vi "Hardware Module.vi"(4 "Light intensity [%]":dbl(ramp), 5 "Mode":enum16{"Ohm", "DcV"}(ring), 6 "write buffer":string, 7 "State":T1(ring), 8 "error in (no error)":errorcluster, 9 "byte count":u32, 10 "baud rate (9600)":u32=9600, 11 "VISA resource name":refnum<visa-resource-name>) -> (0 "error out":errorcluster, 1 "return count":u32, 2 "read buffer":string, 3 "VISA resource name out":refnum<visa-resource-name>)   [LabVIEW 2019]
doc: "Funkcja służy do komunikacji za pomocą portu szeregowergo z multimetrem cyfrowym SANWA PC5000a. Komunikacja odbywa się poprzez bibliotekę NI-VISA z wykorzystaniem podstawowych funkcji portu szeregowego. Funkcja umożliwia emulację hardwaru wówczas jako nazwę urządzenia podać: VirtualDevice1\n\n- VISA resource name specifies the resource to be opened.\n- baud rate is the rate of transmission. The default is 9600. \n- write buffer contains the data to be written to the device. \n- return count contains the actual number of bytes written. \n- State defines the functionality of the function. It contains three values Configure Port, Write, Read and Close\n- Light intensity [%] is used during emulation.\n- error out contains error information. This output provides standard error out functionality.\n\nWięcej pomocy można znaleźć w pomocy funkcji:\nVISA Configure Serial Port VI \nVISA Write Function\nVISA Read Function"
uses:
  <vilib>/Instr/_visa.llb/VISA Configure Serial Port (Instr).vi
  <vilib>/ptbypt/NI_PtbyPt.lvlib
panel:
  # "Inputs"
  # "Outputs"
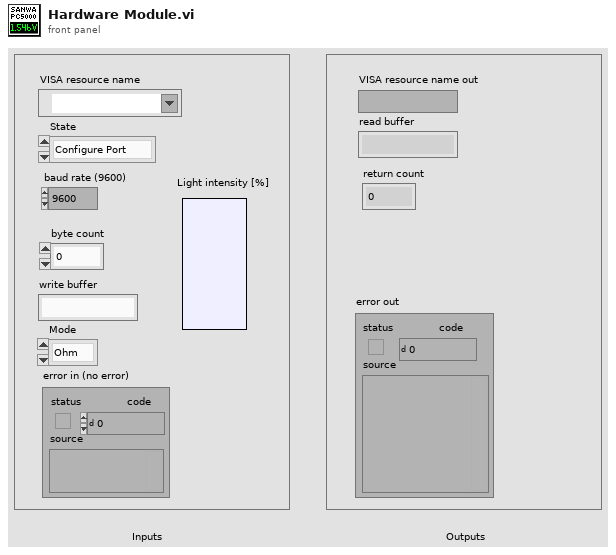
[diagram p1: front panel]
types:
  T1 = enum16{"Configure Port", "Write", "Read", "Close"}
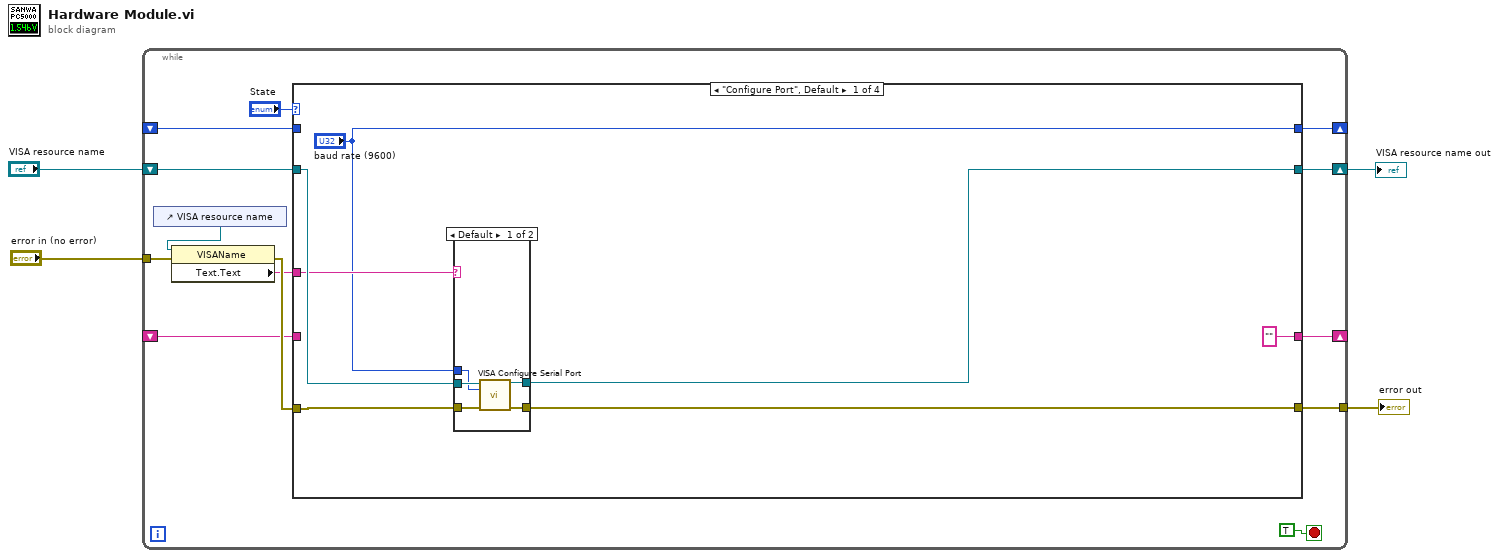
[diagram p0: block diagram]
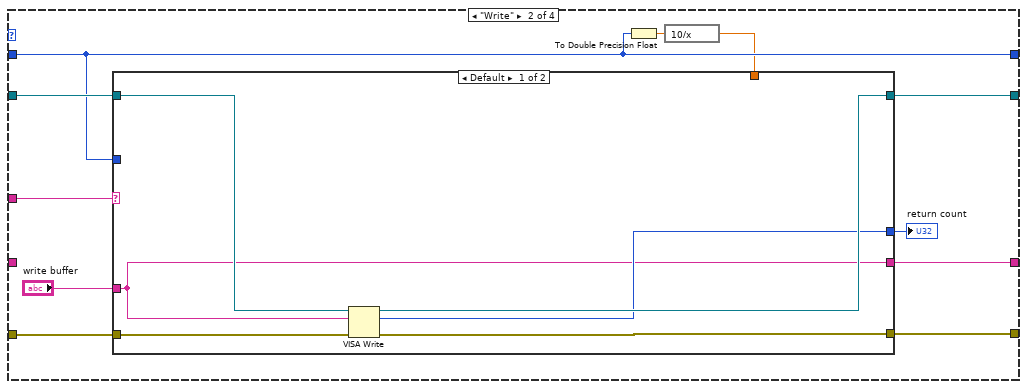
[diagram p3: hidden frame]
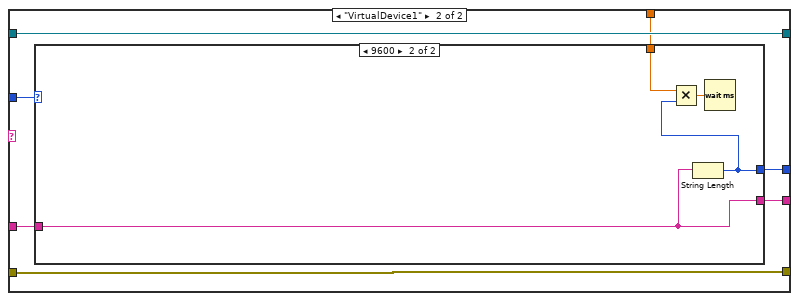
[diagram p4: hidden frame]
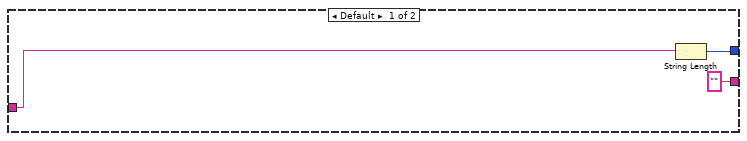
[diagram p5: hidden frame]
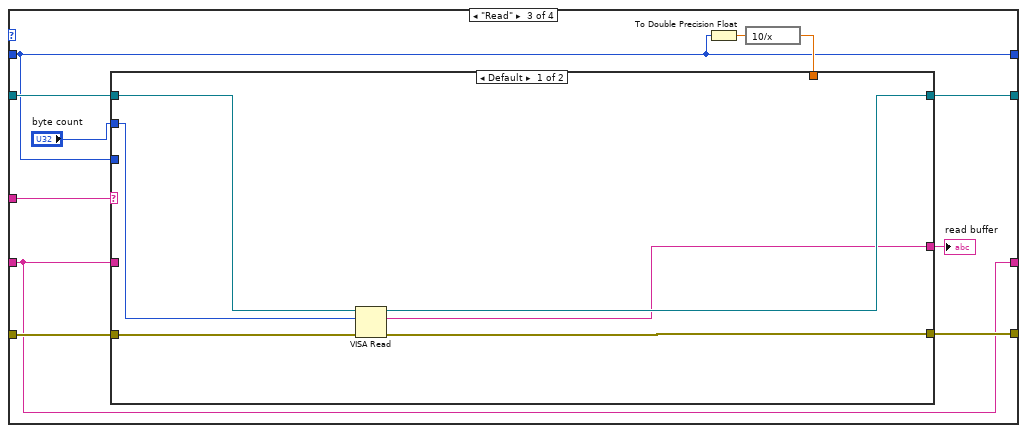
[diagram p6: hidden frame]
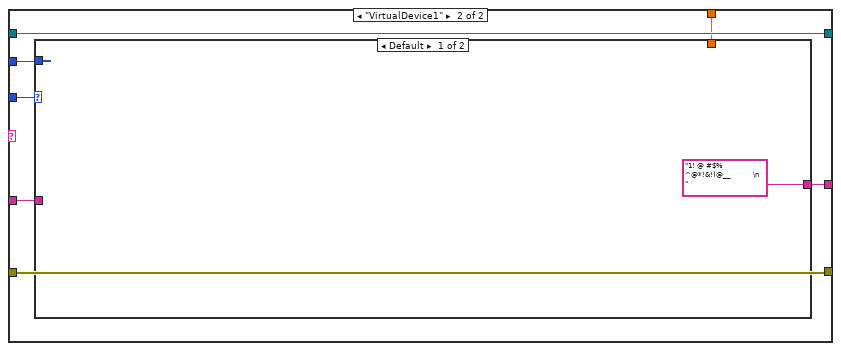
[diagram p7: hidden frame]
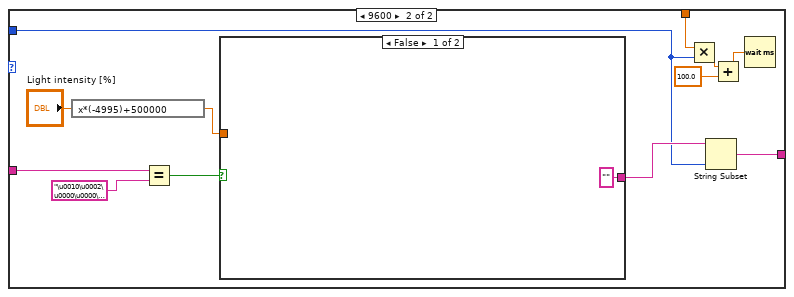
[diagram p8: hidden frame]
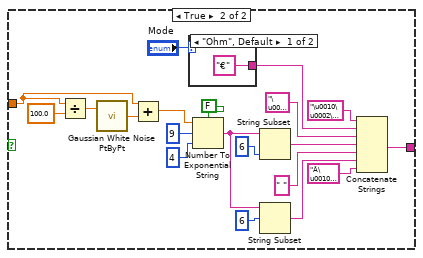
[diagram p9: hidden frame]
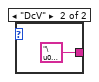
[diagram p10: hidden frame]
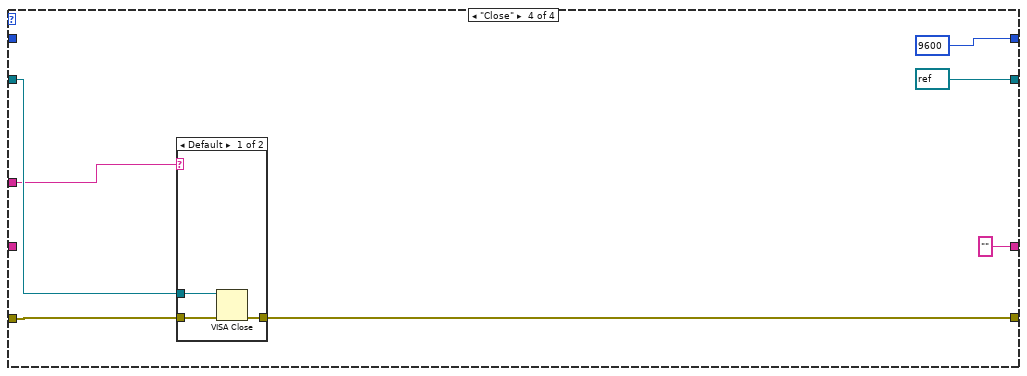
[diagram p11: hidden frame]
diagram:
  n1 = while {
    tunnel: "error in (no error)" -> [w16]
    tunnel: [w14] -> w2
    shift-right: [w15] -> w3
    shift-left: "VISA resource name" -> [w13]
    shift-right: [w11] -> _
    shift-left: _ -> [w8]
    shift-right: [w6] -> _
    shift-left: _ -> [w5]
    stop <- TRUE stop-if-true
    n2 = control-ref of="VISA resource name"() -> (w7:refnum<vi>)
    n3 = property on="Property Node" class="VISAName"(reference=w7, error in=w16) -> (error out=w10:errorcluster, "Text.Text"=w9:string)  [unwired: 1 out]
    n4 = case shown="\"Configure Port\", Default" "State" {
      tunnel: [w24 w38 w73 refnum<visa-resource-name> refnum ("VISA resource name")] -> w15
      tunnel: [w23 w41 w68 w127] -> w14
      tunnel: w13 -> [w22 w40 w72 w128]
      tunnel: ["baud rate (9600)" w34 w64 u32 9600 ("baud rate (9600)")] -> w11
      tunnel: w10 -> [w21 w42 w70 w125]
      tunnel: w9 -> [w20 w39 w71 w126]
      tunnel: w8 -> [_ w34 w64 _]
      tunnel: ["" ("write buffer") w35 w66 "" ("write buffer")] -> w6
      tunnel: w5 -> [_ _ w66 _]
      frame "Configure Port", Default {
        n5 = case shown="Default" w20 {
          tunnel: w21 -> [w29 w31]
          tunnel: [w28 w30] -> w24
          tunnel: [w27 w31] -> w23
          tunnel: w22 -> [w26 w30]
          tunnel: "baud rate (9600)" -> [w25 _]
          frame Default {
            n6 = call-poly "VISA Configure Serial Port"("VISA resource name"=w26, "baud rate (9600)"=w25, "error in (no error)"=w29) -> ("VISA resource name out"=w28:refnum<visa-resource-name>, "error out"=w27:errorcluster)  [unwired: 11 in]
          }
          frame "VirtualDevice1" {
          }
        }
      }
      frame "Write" {
        n7 = To Double Precision Float(number=w34) -> (double precision float=w32:dbl)
        n8 = expression code="10/x"(w32) -> (w33:dbl)
        n9 = case shown="Default" w39 {
          tunnel: w40 -> [w48 w55]
          tunnel: [w45 w49] -> w41
          tunnel: w42 -> [w46 w49]
          tunnel: [w47 w55] -> w38
          tunnel: [w44 w51] -> w37
          tunnel: w34 -> [_ w54]
          tunnel: "write buffer" -> [w43 w52]
          tunnel: [w43 w53] -> w35
          tunnel: w33 -> [_ w50]
          frame Default {
            n10 = VISA Write(VISA resource name=w48, write buffer=w43, error in (no error)=w46) -> (VISA resource name out=w47:refnum<visa-resource-name>, return count=w44:u32, error out=w45:errorcluster)
          }
          frame "VirtualDevice1" {
            n11 = case shown="9600" w54 {
              tunnel: ["" ("write buffer") w62] -> w53
              tunnel: w52 -> [w56 w62]
              tunnel: [w57 w59] -> w51
              tunnel: w50 -> [_ w60]
              frame Default {
                n12 = String Length(string=w56) -> (length=w57:i32)
              }
              frame 9600 {
                n13 = String Length(string=w62) -> (length=w59:i32)
                n14 = Multiply(x=w60, y=w59) -> (x*y=w61:dbl)
                n15 = Wait (ms)(milliseconds to wait=w61) -> ()  [unwired: 1 out]
              }
            }
          }
        }
        "return count" <- w37
      }
      frame "Read" {
        n16 = To Double Precision Float(number=w64) -> (double precision float=w63:dbl)
        n17 = expression code="10/x"(w63) -> (w65:dbl)
        n18 = case shown="Default" w71 {
          tunnel: w72 -> [w79 w86]
          tunnel: [w76 w81] -> w68
          tunnel: w70 -> [w77 w81]
          tunnel: [w78 w86] -> w73
          tunnel: [w75 w83] -> w69
          tunnel: w64 -> [_ w85]
          tunnel: "byte count" -> [w74 w84]
          tunnel: w66 -> [_ w82]
          tunnel: w65 -> [_ w80]
          frame Default {
            n19 = VISA Read(VISA resource name=w79, byte count=w74, error in (no error)=w77) -> (VISA resource name out=w78:refnum<visa-resource-name>, read buffer=w75:string, error out=w76:errorcluster)  [unwired: 1 out]
          }
          frame "VirtualDevice1" {
            n20 = case shown="Default" w85 {
              tunnel: w84 -> [_ w92]
              tunnel: ["1! @ #$%   ^@*!&!)@__           \n                                                               " ("read buffer") w96] -> w83
              tunnel: w82 -> [_ w95]
              tunnel: w80 -> [_ w90]
              frame Default {
              }
              frame 9600 {
                n21 = expression code="x*(-4995)+500000"("Light intensity [%]") -> (w93:dbl)
                n22 = Equal?(x=w95, y="\u0010\u0002\u0000\u0000\u0000\u0000\u0010\u0003" ("string")) -> (x = y?=w98:bool)
                n23 = case shown="False" w98 {
                  tunnel: ["" ("read buffer") w104] -> w97
                  tunnel: w93 -> [_ w119]
                  frame False {
                  }
                  frame True {
                    n24 = Divide(x=w119, y=100.0) -> (x/y=w102:dbl)
                    n25 = call <vilib>:"Gaussian White Noise PtByPt.vi"("standard deviation"=w102) -> ("Gaussian white noise"=w101:dbl)  [unwired: 2 in]
                    n26 = Add(x=w119, y=w101) -> (x+y=w103:dbl)
                    n27 = case shown="\"Ohm\", Default" "Mode" {
                      tunnel: ["€" ("read buffer") "\u0006" ("read buffer")] -> w105
                      frame "Ohm", Default {
                      }
                      frame "DcV" {
                      }
                    }
                    n28 = Number To Exponential String(number=w103, precision (6)=i16 4, 1:FALSE ("use system decimal point (T)"), 3:i16 9 ("width (-)")) -> (E-format string=w113:string)
                    n29 = String Subset(string=w113, length (rest)=6 ("length (rest)")) -> (substring=w112:string)  [unwired: 1 in]
                    n30 = String Subset(string=w113, offset (0)=6 ("length (rest)")) -> (substring=w110:string)  [unwired: 1 in]
                    n31 = Concatenate Strings("\u0010\u0002\u0000\u000f" ("read buffer"), w105, "\u0000\u0000\u0000 " ("read buffer"), w112, " " ("read buffer"), w110, "Â\u0010\u0003" ("read buffer")) -> (w104:string)
                  }
                }
                n32 = Multiply(x=w90, y=w92) -> (x*y=w91:dbl)
                n33 = String Subset(string=w97, length (rest)=w92) -> (substring=w96:string)  [unwired: 1 in]
                n34 = Add(x=w91, y=100.0) -> (x+y=w89:dbl)
                n35 = Wait (ms)(milliseconds to wait=w89) -> ()  [unwired: 1 out]
              }
            }
          }
        }
        "read buffer" <- w69
      }
      frame "Close" {
        n36 = case shown="Default" w126 {
          tunnel: w128 -> [w132 _]
          tunnel: [w131 w133] -> w127
          tunnel: w125 -> [w130 w133]
          frame Default {
            n37 = VISA Close(VISA resource name=w132, error in (no error)=w130) -> (error out=w131:errorcluster)
          }
          frame "VirtualDevice1" {
          }
        }
      }
    }
  }
  "VISA resource name out" <- w3
  "error out" <- w2
